vi "Lezeti_Power_Monitor_18_a.vi"() -> ()   [LabVIEW 2014]
doc: "This example shows how to use autosetup and acquire a waveform on a single channel."
uses:
  <instrlib>/RIGOL DS1000 Series/Public/Data/Read (Multiple Waveforms).vi
  <vilib>/measure/madcrms.llb/Basic Averaged DC-RMS for 1 Chan.vi
  <vilib>/measure/mascope.llb/Cycle Average and RMS 1 chan.vi
  <vilib>/Utility/file.llb/Write To Spreadsheet File (DBL).vi
  <instrlib>/RIGOL DS1000 Series/RIGOL DS1000 Series.lvlib
  <vilib>/measure/NI_MAPro.lvlib
panel:
  out "Power Factor":dbl
  out "Apparent Power (VA)":dbl
  out "Run Date":string
  out "Run Time":string
  out "Elapsed Time (s)":dbl
  in  "Output File":path
  out "Average Power (Watts)":dbl
  out "Instant Power Waveform":waveform(dbl)(graph)
  out "IRMS":dbl
  out "Current Waveform":waveform(dbl)(graph)
  out "VRMS":dbl
  in  "Stop":bool
  out "Voltage Waveform":waveform(dbl)(graph)
  in  "VISA resource name":refnum<visa-resource-name>
  # "For Lezeti Air Conditioning System (Greenpath Tech)\nBy Matsu Thornton\nJuly 2016"
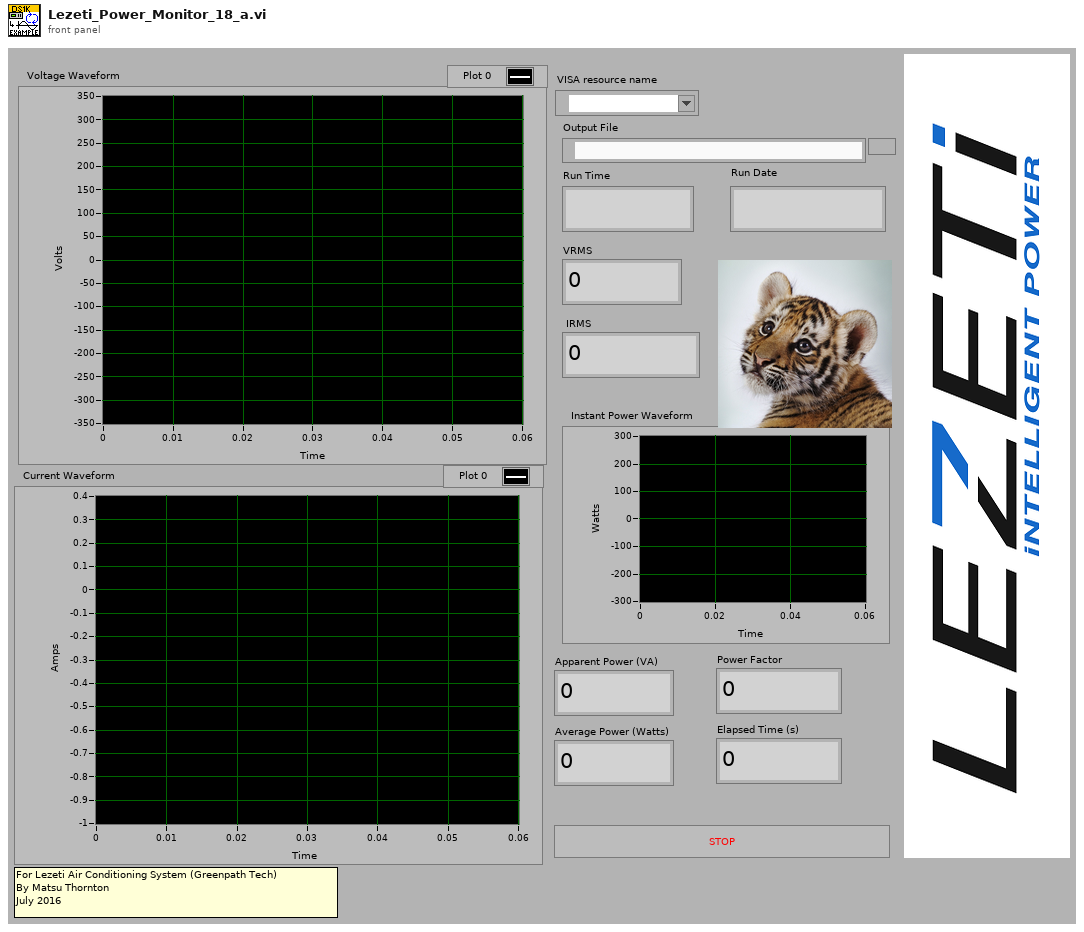
[diagram p1: front panel]
types:
  T1 = typedef "NI_Matrix.lvlib/RealMatrix.ctl" = dbl[][]
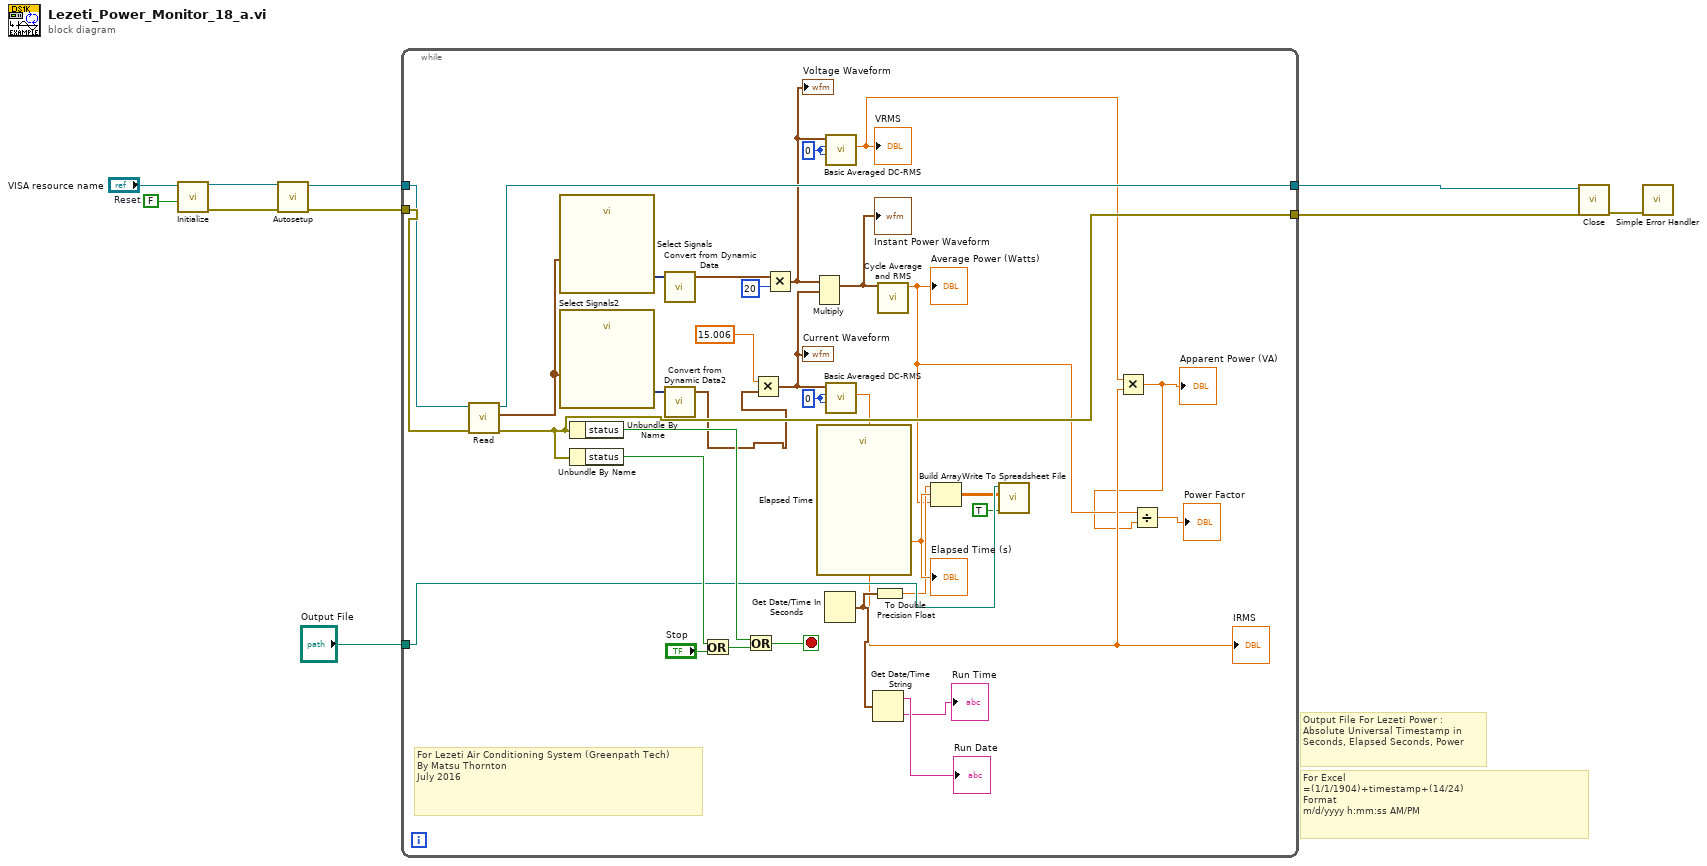
[diagram p0: block diagram]
diagram:
  w3 = FALSE  # Reset
  # "For Excel\n=(1/1/1904)+timestamp+(14/24)\nFormat\nm/d/yyyy h:mm:ss AM/PM"
  # "Output File For Lezeti Power :\nAbsolute Universal Timestamp in Seconds, Elapsed Seconds, Power"
  n1 = call <instrlib>:"Initialize.vi"("Reset (True)"=w3, "VISA resource name"="VISA resource name") -> ("error out"=w7:errorcluster, "VISA resource name out"=w6:refnum<visa-resource-name>)  [unwired: 2 in, 6 out]
  n2 = call <instrlib>:"Autosetup.vi"("error in (no error)"=w7, "VISA resource name"=w6) -> ("error out"=w4:errorcluster, "VISA resource name out"=w5:refnum<visa-resource-name>)  [unwired: 8 out]
  n3 = while {
    tunnel: w5 -> [w24]
    tunnel: w4 -> [w44]
    tunnel: [w43] -> w9
    tunnel: [w25] -> w2
    tunnel: "Output File" -> [w30]
    stop <- w32 stop-if-true
    w38 = 0
    w40 = 0
    # "For Lezeti Air Conditioning System (Greenpath Tech)\nBy Matsu Thornton\nJuly 2016"
    n4 = call-poly <instrlib>:"Read.vi"("error in (no error)"=w44, "VISA resource name"=w24) -> ("error out"=w25:errorcluster, "Waveform Data"=w20:waveform(dbl)[], "VISA resource name out"=w43:refnum<visa-resource-name>)  [unwired: 2 in, 5 out]
    n5 = call "Select Signals"("Signals"=w20) -> ("Signal Out"=w23:dynamicdata)  [unwired: 9 in, 1 out]
    n6 = call "Select Signals2"("Signals"=w20) -> ("Signal Out"=w21:dynamicdata)  [unwired: 9 in, 1 out]
    n7 = Unbundle By Name(w25) -> ("status"=w39:bool)
    n8 = Unbundle By Name(w25) -> ("status"=w42:bool)
    n9 = call "Convert from Dynamic Data"("Dynamic Data Type"=w23) -> ("Waveform"=w22:waveform(dbl))  [unwired: 3 in]
    n10 = call "Convert from Dynamic Data2"("Dynamic Data Type"=w21) -> ("Waveform"=w19:waveform(dbl))  [unwired: 3 in]
    n11 = Or(x=w42, y="Stop") -> (x .or. y?=w33:bool)
    n12 = Or(x=w39, y=w33) -> (x .or. y?=w32:bool)
    n13 = Multiply(x=15.006, y=w19) -> (x*y=w34:waveform(dbl))
    "Current Waveform" <- w34
    n14 = Multiply(x=w22, y=20) -> (x*y=w36:waveform(dbl))
    "Voltage Waveform" <- w36
    n15 = Multiply(1:w34, 2:w36) -> (0:w31:waveform(dbl))  [unwired: 1 in, 1 out]
    "Instant Power Waveform" <- w31
    n16 = call "Elapsed Time"() -> ("Elapsed Time (s)"=w27:dbl)  [unwired: 12 in, 7 out]
    "Elapsed Time (s)" <- w27
    n17 = Get Date/Time In Seconds() -> (seconds since 1Jan1904=w18:timestamp)
    n18 = call-poly <vilib>:"Basic Averaged DC-RMS.vi"("window"=w40, "averaging type"=w40, "signal in"=w36) -> ("RMS value"=w14:dbl)  [unwired: 5 in, 3 out]
    "VRMS" <- w14
    n19 = call-poly <vilib>:"Basic Averaged DC-RMS.vi"("window"=w38, "averaging type"=w38, "signal in"=w34) -> ("RMS value"=w13:dbl)  [unwired: 5 in, 3 out]
    "IRMS" <- w13
    n20 = Get Date/Time String(seconds (now)=w18) -> (date string=→"Run Date":string, time string=→"Run Time":string)  [unwired: 2 in]
    n21 = To Double Precision Float(number=w18) -> (double precision float=w26:dbl)
    n22 = call-poly <vilib>:"Cycle Average and RMS.vi"("signal in"=w31) -> ("cycle average"=w12:dbl)  [unwired: 7 in, 3 out]
    "Average Power (Watts)" <- w12
    n23 = Build Array(w26, w27, w12) -> (w28:T1)
    n24 = call-poly <vilib>:"Write To Spreadsheet File.vi"("append to file? (new file:F)"=TRUE, "2D data"=w28, "file path (dialog if empty)"=w30) -> ()  [unwired: 5 in, 1 out]
    n25 = Multiply(x=w14, y=w13) -> (x*y=w11:dbl)
    "Apparent Power (VA)" <- w11
    n26 = Divide(x=w12, y=w11) -> (x/y=→"Power Factor":dbl)
  }
  n27 = call <instrlib>:"Close.vi"("error in (no error)"=w2, "VISA resource name"=w9) -> ("error out"=w10:errorcluster)  [unwired: 9 out]
  n28 = call <vilib>:"Simple Error Handler.vi"("error in (no error)"=w10) -> ()  [unwired: 1 in, 8 out]
